vi "ScannerTest.vi"(9 "SN":string, 10 "Nth":string, 11 "Station":string) -> ()   [LabVIEW 2020]
uses:
  <vilib>/Utility/config.llb/NI_LVConfig.lvlib
  <vilib>/Utility/config.llb/Read Key (String).vi
panel:
  out "Result":string
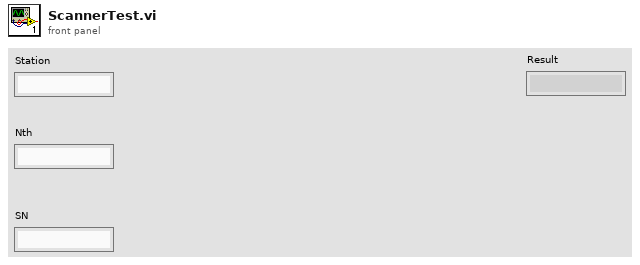
[diagram p1: front panel]
types:
  T1 = typedef "NI_LVConfig.lvlib/Config Data RefNum.ctl" = refnum<k1>
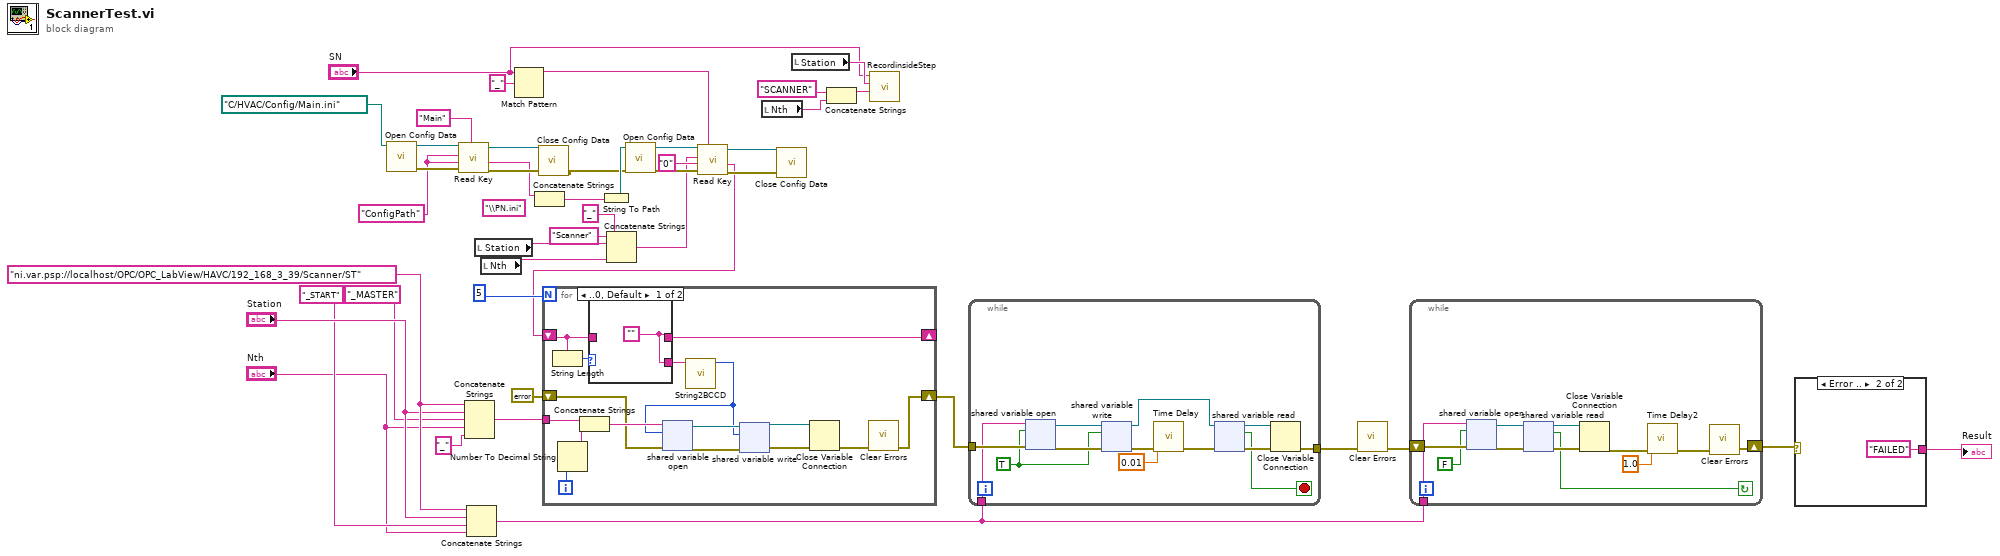
[diagram p0: block diagram]
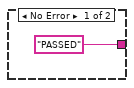
[diagram p2: hidden frame]
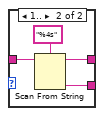
[diagram p3: hidden frame]
diagram:
  w16 = "ni.var.psp://localhost/OPC/OPC_LabView/HAVC/192_168_3_39/Scanner/ST"
  (unwired) "\\PN.ini" ("string")
  w38 = "ConfigPath" ("key")
  n1 = call <vilib>:"Open Config Data.vi"("configuration file path"=path "C:/HVAC/Config/Main.ini") -> ("error out"=w43:errorcluster, "refnum"=w42:T1)  [unwired: 8 in, 1 out]
  n2 = call-poly <vilib>:"Read Key.vi"("section"="Main", "error in (no error)"=w43, "default value"=w38, "key"=w38, "refnum"=w42) -> ("error out"=w40:errorcluster, "value"=w37:string, "refnum out"=w41:T1)  [unwired: 3 in, 1 out]
  n3 = Concatenate Strings(w16, "Station", "_MASTER" ("string"), "Nth", "_" ("string")) -> (w8:string)
  n4 = Concatenate Strings(w16, "Station", "_START" ("string"), "Nth") -> (w5:string)
  n5 = local read "Station"() -> (w19:string)
  n6 = local read "Nth"() -> (w18:string)
  n7 = Match Pattern(string="SN", regular expression="_") -> (before substring=w23:string)  [unwired: 1 in, 3 out]
  n8 = Concatenate Strings(w37) -> (w24:string)  [unwired: 1 in]
  n9 = call <vilib>:"Close Config Data.vi"("error in (no error)"=w40, "refnum"=w41) -> ("error out"=w25:errorcluster)  [unwired: 8 in, 1 out]
  n10 = String To Path(string=w24) -> (path=w26:path)
  n11 = Concatenate Strings("Scanner" ("string"), w19, "_" ("string"), w18) -> (w17:string)
  n12 = call <vilib>:"Open Config Data.vi"("error in (no error)"=w25, "configuration file path"=w26) -> ("error out"=w30:errorcluster, "refnum"=w29:T1)  [unwired: 7 in, 1 out]
  n13 = call-poly <vilib>:"Read Key.vi"("section"=w23, "error in (no error)"=w30, "default value"="0", "key"=w17, "refnum"=w29) -> ("error out"=w27:errorcluster, "value"=w9:string, "refnum out"=w28:T1)  [unwired: 3 in, 1 out]
  n14 = for {
    N: 5 -> [_]
    shift-right: [w60] -> _
    shift-left: w9 -> [w51]
    tunnel: w8 -> [w57]
    shift-right: [w46] -> w7
    shift-left: errorcluster {"status"=FALSE, "code"=0, "source"=""} ("error out") -> [w45]
    i -> [w55]
    n15 = String Length(string=w51) -> (length=w52:i32)
    n16 = Number To Decimal String(number=w55) -> (decimal integer string=w58:string)  [unwired: 1 in]
    n17 = Concatenate Strings(w57, w58) -> (w56:string)
    n18 = case shown="..0, Default" w52 {
      tunnel: w51 -> [_ w65]
      tunnel: [w61 w63] -> w60
      tunnel: [w61 w62] -> w59
      frame ..0, Default {
        w61 = ""
      }
      frame 1.. {
        n19 = Scan From String(format string="%4s", input string=w65) -> (remaining string=w63:string, output 1=w62:string)  [unwired: 3 in, 2 out]
      }
    }
    n20 = call "String2BCCD.vi"("String"=w59) -> ("BCD Int"=w50:i64)  [unwired: 10 in]
    n21 = shared-variable-open(w56, w45, w50) -> (w53:refnum<k21>, w54:errorcluster)  [unwired: 1 in]
    n22 = shared-variable-write(w53, w54, w50) -> (w48:refnum<k21>, w49:errorcluster)
    n23 = Close Variable Connection(8:w49, 11:w48) -> (0:w47:errorcluster)
    n24 = call <vilib>:"Clear Errors.vi"("error in (no error)"=w47) -> ("error out"=w46:errorcluster)  [unwired: 5 in, 1 out]
  }
  n25 = local read "Nth"() -> (w31:string)
  n26 = call <vilib>:"Close Config Data.vi"("error in (no error)"=w27, "refnum"=w28) -> ()  [unwired: 8 in, 2 out]
  n27 = local read "Station"() -> (w35:string)
  n28 = Concatenate Strings("SCANNER", w31) -> (w33:string)
  n29 = call "RecordinsideStep.vi"("STEP"=w33, "Station"=w35, "SN"="SN") -> ()  [unwired: 8 in, 1 out]
  n30 = while {
    tunnel: w7 -> [w76]
    tunnel: w5 -> [w75]
    tunnel: [w66] -> w4
    stop <- w67 stop-if-true
    w74 = TRUE
    n31 = shared-variable-open(w75, w76, w74) -> (w77:refnum<k21>, w78:errorcluster)  [unwired: 1 in]
    n32 = shared-variable-write(w77, w78, w74) -> (w68:refnum<k21>, w73:errorcluster)
    n33 = call "Time Delay"("error in (no error)"=w73, "Delay Time (s)"=0.01) -> ("error out"=w70:errorcluster)  [unwired: 9 in]
    n34 = shared-variable-read(w68, w70) -> (w69:refnum<k21>, w71:errorcluster, w67:bool)  [unwired: 1 out]
    n35 = Close Variable Connection(8:w71, 11:w69) -> (0:w66:errorcluster)
  }
  n36 = call <vilib>:"Clear Errors.vi"("error in (no error)"=w4) -> ("error out"=w3:errorcluster)  [unwired: 5 in, 1 out]
  n37 = while {
    tunnel: w5 -> [w89]
    shift-right: [w79] -> w1
    shift-left: w3 -> [w90]
    stop <- w84 continue-if-true
    n38 = shared-variable-open(w89, w90, FALSE) -> (w83:refnum<k21>, w82:errorcluster)  [unwired: 1 in]
    n39 = shared-variable-read(w83, w82) -> (w85:refnum<k21>, w86:errorcluster, w84:bool)  [unwired: 1 out]
    n40 = Close Variable Connection(8:w86, 11:w85) -> (0:w81:errorcluster)
    n41 = call "Time Delay2"("error in (no error)"=w81, "Delay Time (s)"=1.0) -> ("error out"=w80:errorcluster)  [unwired: 9 in]
    n42 = call <vilib>:"Clear Errors.vi"("error in (no error)"=w80) -> ("error out"=w79:errorcluster)  [unwired: 5 in, 1 out]
  }
  n43 = case shown="Error .." w1 {
    tunnel: ["PASSED" "FAILED"] -> w2
    frame No Error {
    }
    frame Error {
    }
  }
  "Result" <- w2
